vi "GF_AddKeyedStringToLog.vi"(1 "Value String":string, 2 "Key Name":string, 3 "Current Log":string) -> (0 "concatenated string":string)   [LabVIEW 2016]
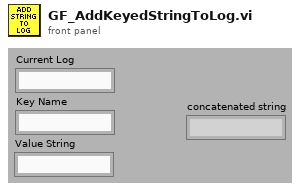
[diagram p1: front panel]
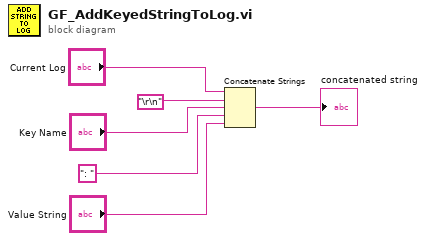
[diagram p0: block diagram]
diagram:
  n1 = Concatenate Strings("Current Log", "\r\n", "Key Name", ": " ("string"), "Value String") -> (→"concatenated string":string)
